vi "CCSendDCMFile.vi"() -> (3 "ResultStatus":i32(ring) items=["Success", "Cancel", "Pending", "Warning", "Failure"])   [LabVIEW 2013, in "main.lvlib" / "ClearCanvasLibrary.lvlib"]
uses:
  ClearCanvasLibrary.lvlib
  C:/Users/Simon/SkyDrive/LabView/2013/DM2020/DICOM/ClearCanvasNewBuild/ClearCanvas.Dicom.dll
  ClearCanvasNewBuild/ClearCanvas.Dicom.dll
panel:
  in  "remotePort":i32=104
  in  "remoteHost":string="www.dicomserver.co.uk"
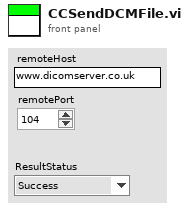
[diagram p1: front panel]
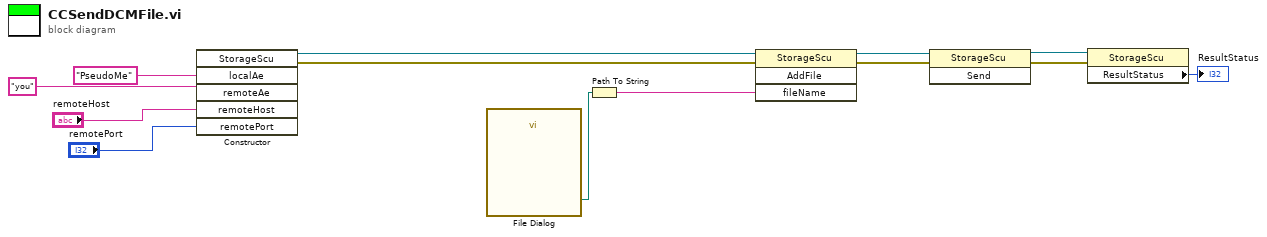
[diagram p0: block diagram]
diagram:
  n1 = constructor class="StorageScu"("localAe"="PseudoMe", "remoteAe"="you", "remoteHost"="remoteHost", "remotePort"="remotePort") -> (reference out=w2:refnum<k24>, error out=w3:errorcluster)  [unwired: 3 in, 5 out]
  n2 = call "File Dialog"() -> ("selected path"=w6:path)  [unwired: 12 in, 3 out]
  n3 = Path To String(path=w6) -> (string=w1:string)
  n4 = invoke class="StorageScu" method="AddFile"(reference=w2, error in=w3, "fileName"=w1) -> (reference out=w5:refnum<k24>, error out=w4:errorcluster)  [unwired: 1 in, 2 out]
  n5 = invoke class="StorageScu" method="Send"(reference=w5, error in=w4) -> (reference out=w11:refnum<k24>, error out=w13:errorcluster)  [unwired: 1 in, 1 out]
  n6 = property class="StorageScu"(reference=w11, error in=w13) -> ("ResultStatus"=→"ResultStatus":i32)  [unwired: 2 out]
